vi "mono_send_vehicle_command.vi"(4 "error in (no error)":errorcluster, 5 "TCP Network Connection in":refnum<k5>, 6 "right_amount":dbl, 7 "forward_amount":dbl) -> (0 "error out":errorcluster, 1 "TCP Network Connection out":refnum<k5>, 3 "vehicle command response 2":string)   [LabVIEW 2018, in "monoDrive.lvlib"]
uses:
  monoDrive.lvlib
  mono_commands.ctl
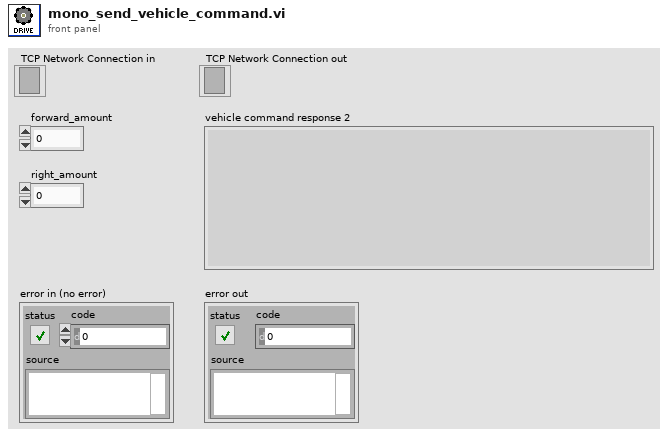
[diagram p1: front panel]
types:
  T1 = cluster{"type":string, "success":bool, "message":cluster{"forward_amount":dbl, "right_amount":dbl}}
  T2 = typedef "monoDrive.lvlib/mono_commands.ctl" = cluster{"SIMULATOR_STATUS_UUID":string, "STREAM_DATA_COMMAND_UUID":string, "SIMULATOR_CONFIG_COMMAND_UUID":string, "VEHICLE_CONFIG_COMMAND_UUID":string, "EGO_CONTROL_COMMAND_UID":string, "WAYPOINT_UPDATE_COMMAND_UID":string, "SCENARIO_COMMAND_UID":string, "MAP_COMMAND_UID":string, "SPAWN_COMMAND_UID":string, "MOVE_ACTOR_COMMAND_UID":string, "SCENARIO_INIT_COMMAND_UID":string, "ATTACH_SENSOR_COMMAND_UID":string, "DETACH_SENSOR_COMMAND_UID":string, "CONTROL_HEADER":string, "RESPONSE_HEADER":string}
  T3 = cluster{"forward_amount":dbl, "right_amount":dbl}
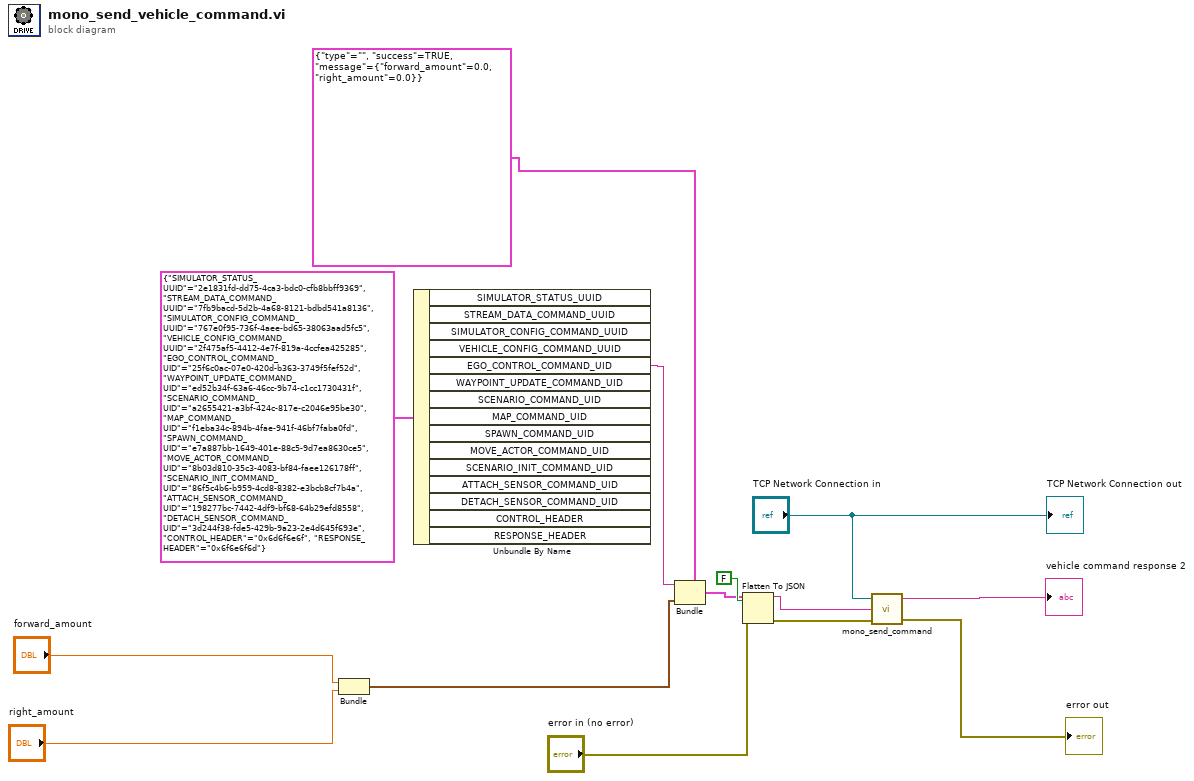
[diagram p0: block diagram]
diagram:
  n1 = Bundle("forward_amount"="forward_amount", "right_amount"="right_amount") -> (w1:T3)  [unwired: 1 in]
  n2 = Unbundle By Name(T2 {"SIMULATOR_STATUS_UUID"="2e1831fd-dd75-4ca3-bdc0-cfb8bbff9369", "STREAM_DATA_COMMAND_UUID"="7fb9bacd-5d2b-4a68-8121-bdbd541a8136", "SIMULATOR_CONFIG_COMMAND_UUID"="767e0f95-736f-4aee-bd65-38063aad5fc5", "VEHICLE_CONFIG_COMMAND_UUID"="2f475af5-4412-4e7f-819a-4ccfea425285", "EGO_CONTROL_COMMAND_UID"="25f6c0ac-07e0-420d-b363-3749f5fef52d", "WAYPOINT_UPDATE_COMMAND_UID"="ed52b34f-63a6-46cc-9b74-c1cc1730431f", "SCENARIO_COMMAND_UID"="a2655421-a3bf-424c-817e-c2046e95be30", "MAP_COMMAND_UID"="f1eba34c-894b-4fae-941f-46bf7faba0fd", "SPAWN_COMMAND_UID"="e7a887bb-1649-401e-88c5-9d7ea8630ce5", "MOVE_ACTOR_COMMAND_UID"="8b03d810-35c3-4083-bf84-faee126178ff", "SCENARIO_INIT_COMMAND_UID"="86f5c4b6-b959-4cd8-8382-e3bcb8cf7b4a", "ATTACH_SENSOR_COMMAND_UID"="198277bc-7442-4df9-bf68-64b29efd8558", "DETACH_SENSOR_COMMAND_UID"="3d244f38-fde5-429b-9a23-2e4d645f693e", "CONTROL_HEADER"="0x6d6f6e6f", "RESPONSE_HEADER"="0x6f6e6f6d"} ("Cluster")) -> ("EGO_CONTROL_COMMAND_UID"=w8:string)  [unwired: 14 out]
  n3 = Bundle(cluster=T1 {"type"="", "success"=TRUE, "message"={"forward_amount"=0.0, "right_amount"=0.0}}, "type"=w8, "message"=w1) -> (w5:T1)  [unwired: 1 in]
  n4 = Flatten To JSON(enable LabVIEW extensions? (T)=FALSE, anything=w5, error in (no error)="error in (no error)") -> (JSON string=w4:string, 11:w12:errorcluster)
  n5 = call "mono_send_command.vi"("error in (no error)"=w12, "JSON Command"=w4, "TCP Network Connection in"="TCP Network Connection in") -> ("error out"=→"error out":errorcluster, "response"=→"vehicle command response 2":string)  [unwired: 1 in]
  "TCP Network Connection out" <- "TCP Network Connection in"
